vi "NewDataInBuffer_Name.vi"() -> (1 "MessageName":string)   [LabVIEW 2017, in "DataAccumulator.lvlib"]
uses:
  <vilib>/addons/InsightCM/Devices/Shared/Common/DataAccumulator/DataAccumulator.lvlib
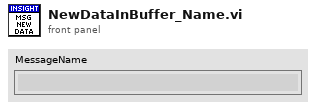
[diagram p1: front panel]
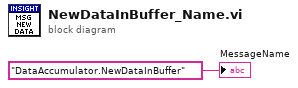
[diagram p0: block diagram]
diagram:
  "MessageName" <- "DataAccumulator.NewDataInBuffer" ("ProcessName")
